vi "WRITE PORT COMvi.vi"(10 "CANAL":u8) -> (1 "BYTES EXPECTED":i32, 2 "COMANDO":string, 3 "EXPECTED RESPONSE":string)   [LabVIEW 2019, in "SERIAL DEVICE.lvclass"]
uses:
  SERIAL DEVICE.lvclass
  COMANDOS.ctl
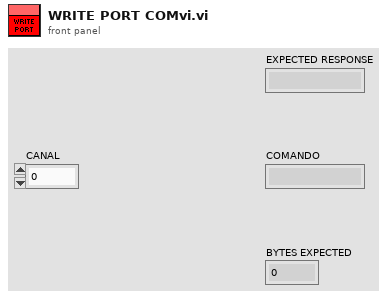
[diagram p1: front panel]
types:
  T1 = typedef "COMANDOS.ctl" = string
  T2 = typedef "MICROS.ctl" = string
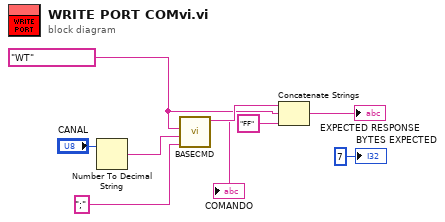
[diagram p0: block diagram]
diagram:
  w5 = T1 "WT" ("COMANDOS")
  n1 = Number To Decimal String(number="CANAL") -> (decimal integer string=w8:string)  [unwired: 1 in]
  n2 = call "BASECMD.vi"("PARÁMETRO 2"=";", "PARÁMETRO 1"=w8, "COMANDOS"=w5) -> ("COMANDO"=→"COMANDO":string, "MICROS"=w6:T2)  [unwired: 7 in]
  n3 = Concatenate Strings(w6, w5, "FF") -> (→"EXPECTED RESPONSE":string)
  "BYTES EXPECTED" <- 7 ("BYTES EXPECTED")
